vi "Actor Core.vi"(8 "error in":errorcluster, 11 "TopLevelApplication In":refnum<class "ConcreteViewModel.lvclass">) -> (0 "error out":errorcluster, 3 "Actor out":refnum<class "Actor.lvclass">)   [LabVIEW 2015, in "TopLevelApplication.lvlib" / "ConcreteViewModel.lvclass"]
doc: "(<B>Filename</B>: Actor Framework.lvlib:Actor.lvclass:Actor Core.vi)\n\nReceives messages to the actor, reacts to them, and initiates any error handling that may shut the actor down.\n\nDescendant classes may override this VI to append parallel tasks for the actor to complete while it handles messages. Overrides use the Call Parent Method node.\n\n<License>\nCopyright © 2017 Composed Systems, LLC | All rights reserved\nwww.composed.io\n\nAuthor: Ethan Stern <ethan.stern@composed.io>\n\nThis software is provided \"AS IS\" WITHOUT WARRANTIES, either express or implied, AND IS FOR EDUCATIONAL PURPOSES ONLY.\n</License>"
uses:
  ConcreteViewModel.lvclass
  <vilib>/ActorFramework/Actor/Actor.lvclass
  Framework/IViewModel/IViewModel/IViewModel.lvclass/IViewModel.ctl
  <vilib>/ActorFramework/Actor/Actor.lvclass/Actor.ctl
  <vilib>/ActorFramework/Message Enqueuer/Message Enqueuer.lvclass/Message Enqueuer.ctl
  Framework/AutoRegistration/ActorAutoRegistration/ActorAutoRegistration.lvclass/ActorAutoRegistration.ctl
  <vilib>/ActorFramework/Message Enqueuer/Init from Existing Queue.vi
  Libraries/ProtectedSubpanel.lvlibp/New Protected Subpanel.vi
  Framework/AutoRegistration/AutoRegistration/Register for Panel Events.vi
  <vilib>/ActorFramework/Message Enqueuer/Message Enqueuer.lvclass
  Framework/AutoRegistration/ActorAutoRegistration/ActorAutoRegistration.lvclass
  Framework/IViewModel/IViewModel/IViewModel.lvclass
panel:
  # "User-defined concrete Model Actor -- All UI stuff happens in the main subpanel\n(over this comment)"
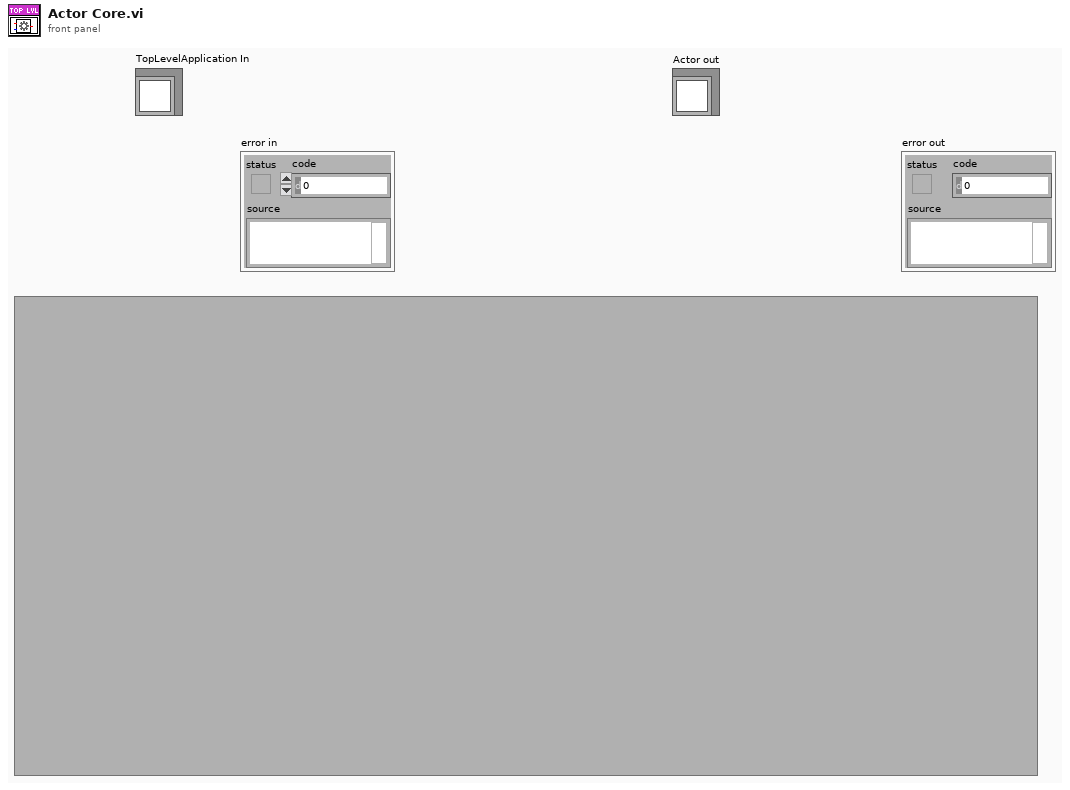
[diagram p1: front panel]
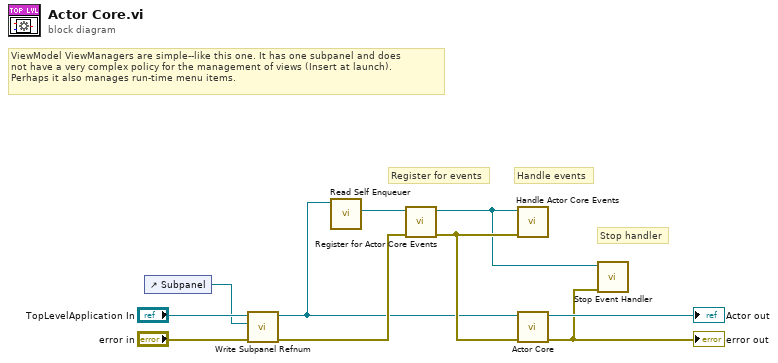
[diagram p0: block diagram]
diagram:
  # "Stop handler"
  # "Handle events"
  # "Register for events"
  # "ViewModel ViewManagers are simple--like this one. It has one subpanel and does\nnot have a very complex policy for the management of views (Insert at launch).\nPerhaps it also manages run-time menu items."
  n1 = control-ref of="Subpanel"() -> (w7:refnum<vi>)
  n2 = call "Write Subpanel Refnum.vi"("error in (no error)"="error in", "SubPnl Refnum"=w7, "IViewModel In"="TopLevelApplication In") -> ("error out"=w6:errorcluster, "IViewModel Out"=w1:refnum<class "ConcreteViewModel.lvclass">)  [unwired: 7 in]
  n3 = call <vilib>:"Read Self Enqueuer.vi"("Actor"=w1) -> ("Self Enqueuer"=w2:refnum<class "Message Enqueuer.lvclass">)  [unwired: 10 in]
  n4 = call "Register for Actor Core Events.vi"("error in (no error)"=w6, "Actor Enqueuer"=w2) -> ("error out"=w5:errorcluster, "ActorAutoRegistration Out"=w4:refnum<class "ActorAutoRegistration.lvclass">)  [unwired: 8 in]
  n5 = call-dynamic "Handle Actor Core Events.vi"("error in (no error)"=w5, "ActorAutoRegistration"=w4) -> ()  [unwired: 9 in, 1 out]
  n6 = call-parent "Actor Core.vi"("error in"=w5, "IViewModel In"=w1) -> ("error out"=w3:errorcluster, "Actor out"=→"Actor out":refnum<class "Actor.lvclass">)  [unwired: 8 in]
  "error out" <- w3
  n7 = call-dynamic "Stop Event Handler.vi"("error in (no error)"=w3, "ActorAutoRegistration In"=w4) -> ()  [unwired: 9 in, 1 out]
